vi "Configure.vi"(8 "error in (no error)":errorcluster, 11 "Harmonics in":refnum<class "Harmonics.lvclass">) -> (0 "error out":errorcluster, 3 "Harmonics out":refnum<class "Harmonics.lvclass">)   [LabVIEW 2020, in "Harmonics.lvclass"]
doc: "Configure the measurements paramaters to sweep.\nThis should be a pop up interface invoked by the configure test button on the main panel."
uses:
  Harmonics.lvclass
  Controls/Loop order.ctl
  Harmonics.lvclass/Harmonics.ctl
  Controls/Config info.ctl
panel:
  in  "Stop level":dbl=999.0 caption="Stop if harmonics higher than (dBm)"
  in  "Zero span":bool
  in  "Use PM for power leveling":bool
  in  "Power (dBm)":string="-40:-30/2"
  in  "Frequency (MHz)":string="900"
  in  "Power Meter number":u8=1
  in  "Power Window":dbl
  in  "Loop order":T1
  in  "All up to Spectrum Analyzer max frequency?":bool
  in  "OK Button":bool
  in  "Average On":bool
  in  "Number of Averages":i32=1 min=0 step=1
  in  "VBW (Hz)":dbl format="%#_6p"
  in  "RBW (Hz)":dbl format="%#_6p"
  in  "Harmonics to Measure":i32(listbox)
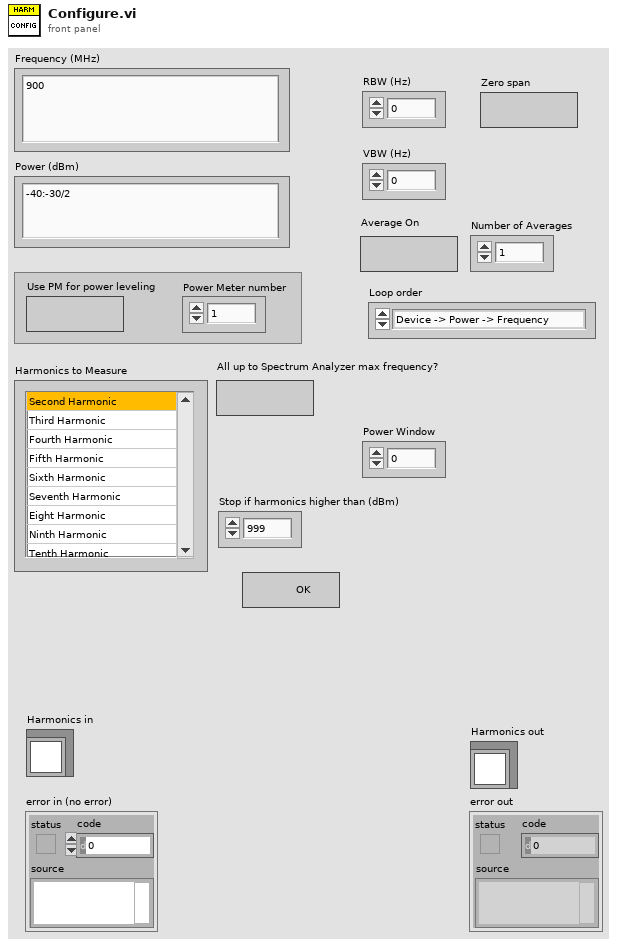
[diagram p1: front panel]
types:
  T1 = typedef "Harmonics.lvclass/Loop order.ctl" = enum16{"Device -> Power -> Frequency", "Device -> Frequency -> Power"}
  T2 = enum8{"Enabled", "Disabled", "Disabled and Grayed Out"}
  T3 = typedef "Harmonics.lvclass/Config info.ctl" = cluster{"RBW":dbl, "VBW ":dbl, "Number of Averages":i32, "Average On":bool, "Symbols":i32[], "All Harm":bool, "Loop order":T1, "Power Window":dbl, "Frequency (MHz)":string, "Power (dBm)":string, "PM for power leveling":u8, "Zero span":bool, "Stop level":dbl}
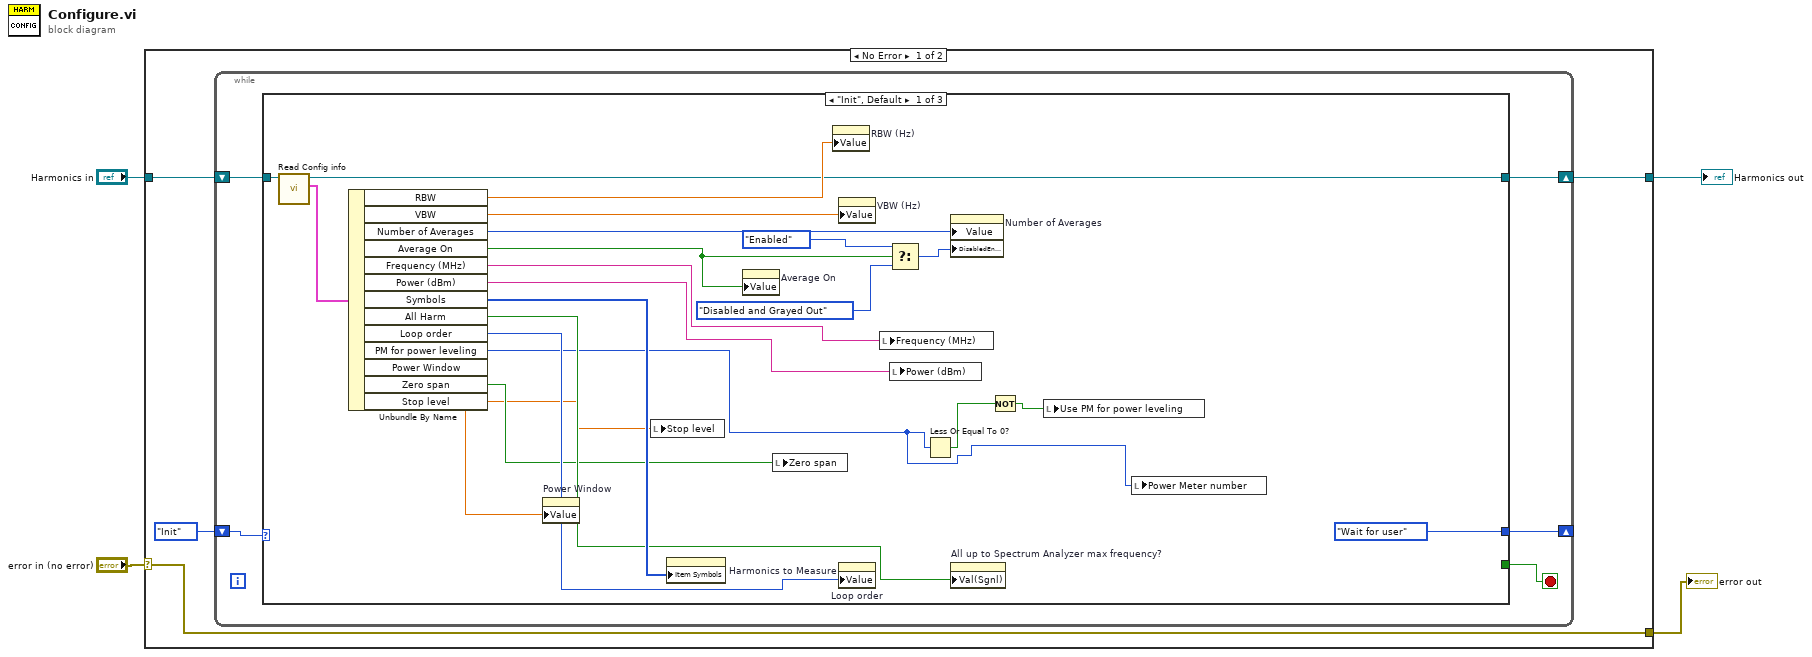
[diagram p0: block diagram]
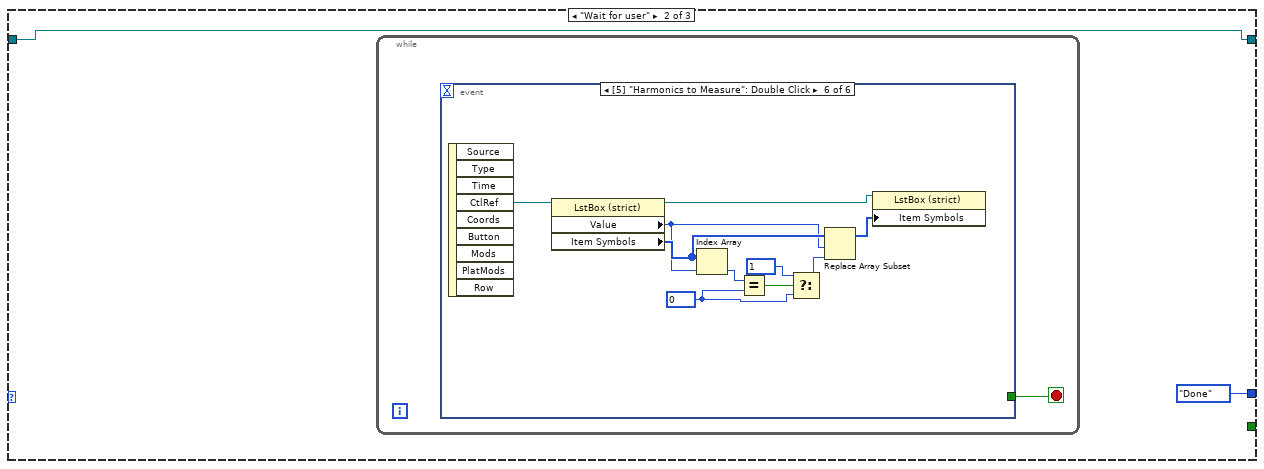
[diagram p2: hidden frame]
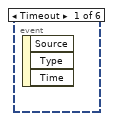
[diagram p3: hidden frame]
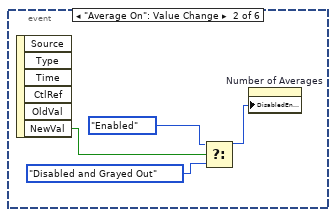
[diagram p4: hidden frame]
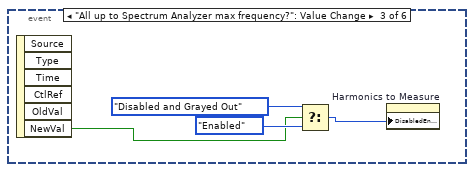
[diagram p5: hidden frame]
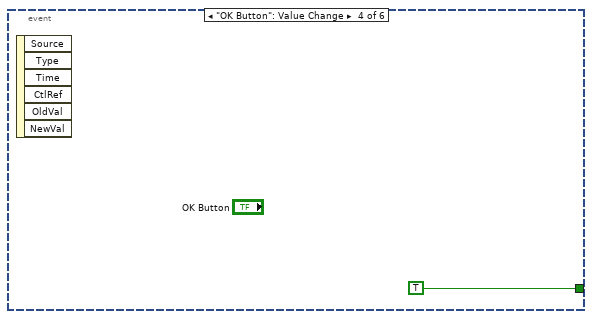
[diagram p6: hidden frame]
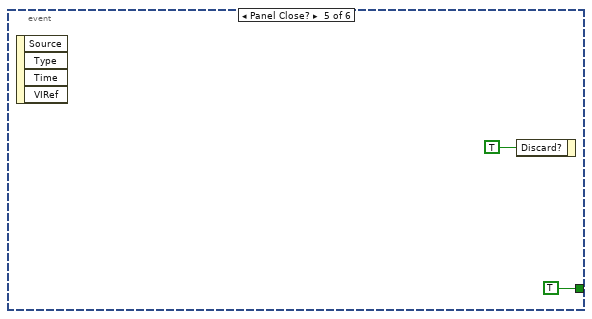
[diagram p7: hidden frame]
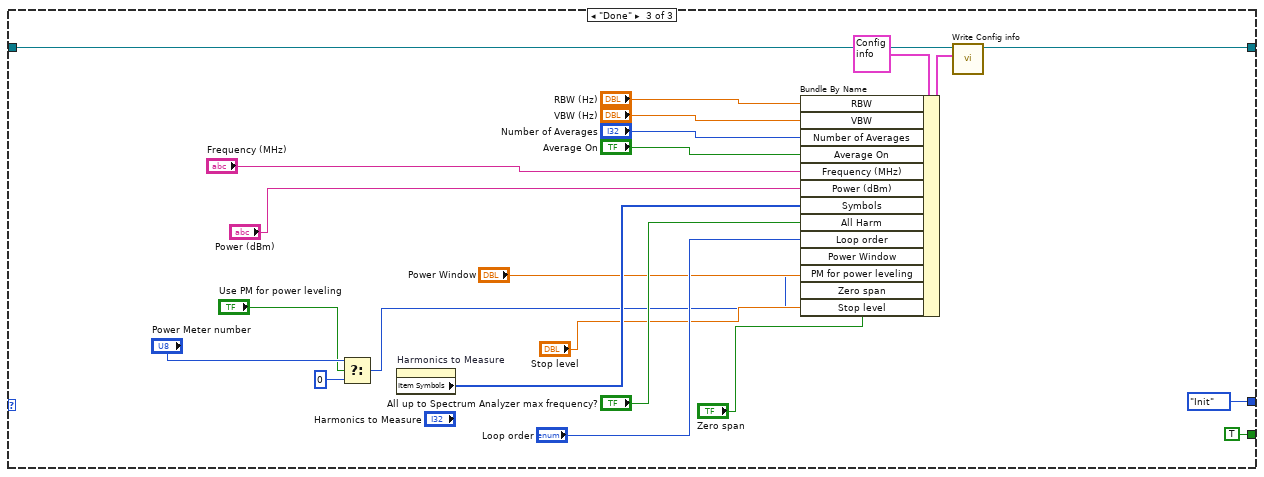
[diagram p8: hidden frame]
diagram:
  n1 = case shown="No Error" "error in (no error)" {
    selector: "error in (no error)" -> [w5 w82]
    tunnel: "Harmonics in" -> [w8 w83]
    tunnel: [w7 w83] -> w2
    tunnel: [w5 w82] -> w1
    frame No Error {
      n2 = while {
        shift-right: [w12] -> w7
        shift-left: w8 -> [w13]
        shift-right: [w10] -> _
        shift-left: enum16{"Init", "Wait for user", "Done"}."Init" -> [w11]
        stop <- w9 stop-if-true
        n3 = case shown="\"Init\", Default" w11 {
          tunnel: w13 -> [w35 w37 w78]
          tunnel: [w26 w37 w79] -> w12
          tunnel: [enum16{"Init", "Wait for user", "Done"}."Wait for user" enum16{"Init", "Wait for user", "Done"}."Done" enum16{"Init", "Wait for user", "Done"}."Init"] -> w10
          tunnel: [_ _ TRUE] -> w9
          frame "Init", Default {
            n4 = call "Read Config info.vi"("Harmonics in"=w35) -> ("Config info"=w34:T3, "Harmonics out"=w26:refnum<class "Harmonics.lvclass">)  [unwired: 9 in]
            n5 = Unbundle By Name(w34) -> ("RBW"=w33:dbl, "VBW"=w32:dbl, "Number of Averages"=w22:i32, "Average On"=w28:bool, "Frequency (MHz)"=w20:string, "Power (dBm)"=w19:string, "Symbols"=w27:i32[], "All Harm"=w24:bool, "Loop order"=w23:T1, "PM for power leveling"=w14:u8, "Power Window"=w21:dbl, "Zero span"=w18:bool, "Stop level"=w17:dbl)
            n6 = property on="Power Window" class="DigNum (strict)"("Value"=w21) -> ()  [unwired: 2 in, 2 out]
            n7 = local write "Stop level"(w17) -> ()
            n8 = property on="Harmonics to Measure" class="LstBox (strict)"("Item Symbols"=w27) -> ()  [unwired: 2 in, 2 out]
            n9 = property on="Average On" class="Bool (strict)"("Value"=w28) -> ()  [unwired: 2 in, 2 out]
            n10 = local write "Zero span"(w18) -> ()
            n11 = property on="RBW (Hz)" class="DigNum (strict)"("Value"=w33) -> ()  [unwired: 2 in, 2 out]
            n12 = property on="VBW (Hz)" class="DigNum (strict)"("Value"=w32) -> ()  [unwired: 2 in, 2 out]
            n13 = property on="Loop order" class="Enum (strict)"("Value"=w23) -> ()  [unwired: 2 in, 2 out]
            n14 = local write "Frequency (MHz)"(w20) -> ()
            n15 = Select(t=T2."Enabled" ("Disabled"), s=w28, f=T2."Disabled and Grayed Out") -> (s? t:f=w30:T2)
            n16 = local write "Power (dBm)"(w19) -> ()
            n17 = Less Or Equal To 0?(x=w14) -> (x <= 0?=w16:bool)
            n18 = property on="Number of Averages" class="DigNum (strict)"("Value"=w22, "DisabledEnum"=w30) -> ()  [unwired: 2 in, 2 out]
            n19 = property on="All up to Spectrum Analyzer max frequency?" class="Bool (strict)"("Val(Sgnl)"=w24) -> ()  [unwired: 2 in, 2 out]
            n20 = Not(x=w16) -> (.not. x?=w15:bool)
            n21 = local write "Use PM for power leveling"(w15) -> ()
            n22 = local write "Power Meter number"(w14) -> ()
          }
          frame "Wait for user" {
            n23 = while {
              stop <- w38 stop-if-true
              n24 = event shown="[5] \"Harmonics to Measure\": Double Click" {
                selector: _ -> [_ _ _ _ _ _]
                dyn-events: _ -> [_ _ _ _ _ _]
                timeout: _ -> [_ _ _ _ _ _]
                tunnel: [_ _ _ TRUE TRUE _] -> w38
                event Timeout {
                  n25 = event-data() -> ()  [unwired: 1 in, 3 out]
                }
                event "Average On": Value Change {
                  n26 = event-data() -> ("NewVal"=w42:bool)  [unwired: 1 in, 5 out]
                  n27 = Select(t=T2."Enabled" ("Disabled"), s=w42, f=T2."Disabled and Grayed Out" ("Disabled")) -> (s? t:f=w41:T2)
                  n28 = property on="Number of Averages" class="DigNum (strict)"("DisabledEnum"=w41) -> ()  [unwired: 2 in, 2 out]
                }
                event "All up to Spectrum Analyzer max frequency?": Value Change {
                  n29 = event-data() -> ("NewVal"=w43:bool)  [unwired: 1 in, 5 out]
                  n30 = Select(t=T2."Disabled and Grayed Out", s=w43, f=T2."Enabled" ("Disabled")) -> (s? t:f=w44:T2)
                  n31 = property on="Harmonics to Measure" class="LstBox (strict)"("DisabledEnum"=w44) -> ()  [unwired: 2 in, 2 out]
                }
                event "OK Button": Value Change {
                  n32 = event-data() -> ()  [unwired: 1 in, 6 out]
                }
                event Panel Close? {
                  n33 = event-data() -> ()  [unwired: 1 in, 4 out]
                  n34 = event-data("Discard?"=TRUE) -> ()  [unwired: 1 in, 1 out]
                }
                event "Harmonics to Measure": Double Click {
                  w56 = 0
                  n35 = event-data() -> ("CtlRef"=w59:refnum<vi>)  [unwired: 1 in, 8 out]
                  n36 = property class="LstBox (strict)"(reference=w59) -> (reference out=w51:refnum<vi>, "Value"=w52:i32, "Item Symbols"=w53:i32[])  [unwired: 1 in, 1 out]
                  n37 = Index Array(array=w53, index=w52) -> (element=w58:i32)
                  n38 = Equal?(x=w58, y=w56) -> (x = y?=w57:bool)
                  n39 = Select(t=1, s=w57, f=w56) -> (s? t:f=w54:i32)
                  n40 = Replace Array Subset(array=w53, new element=w54, index=w52) -> (w50:i32[])
                  n41 = property class="LstBox (strict)"(reference=w51, "Item Symbols"=w50) -> ()  [unwired: 1 in, 2 out]
                }
              }
            }
          }
          frame "Done" {
            n42 = Select(t="Power Meter number", s="Use PM for power leveling", f=u8 0) -> (s? t:f=w61:u8)
            n43 = property on="Harmonics to Measure" class="LstBox (strict)"() -> ("Item Symbols"=w73:i32[])  [unwired: 2 in, 2 out]
            n44 = Bundle By Name(cluster=T3 {"RBW"=0.0, "VBW "=0.0, "Number of Averages"=0, "Average On"=FALSE, "Symbols"=[], "All Harm"=FALSE, "Loop order"=enum."Device -> Power -> Frequency", "Power Window"=0.0, "Frequency (MHz)"="900", "Power (dBm)"="-40:-30/2", "PM for power leveling"=0, "Zero span"=FALSE, "Stop level"=999.0} ("Config info"), "RBW"="RBW (Hz)", "VBW"="VBW (Hz)", "Number of Averages"="Number of Averages", "Average On"="Average On", "Frequency (MHz)"="Frequency (MHz)", "Power (dBm)"="Power (dBm)", "Symbols"=w73, "All Harm"="All up to Spectrum Analyzer max frequency?", "Loop order"="Loop order", "Power Window"="Power Window", "PM for power leveling"=w61, "Zero span"="Zero span", "Stop level"="Stop level") -> (w70:T3)
            n45 = call "Write Config info.vi"("Config info"=w70, "Harmonics in"=w78) -> ("Harmonics out"=w79:refnum<class "Harmonics.lvclass">)  [unwired: 9 in]
          }
        }
      }
    }
    frame Error {
    }
  }
  "error out" <- w1
  "Harmonics out" <- w2
